vi "Eight 8-bit Ports Digital Output.vi"(2 "Packet":u64, 4 "Four 8-bit DO Ports":T1={"8-bit DO Port0"="Chassis1/Mod3/DO7:0", "8-bit DO Port1"="Chassis1/Mod3/DO7:0", "8-bit DO Port2"="Chassis1/Mod3/DO7:0", "8-bit DO Port3"="Chassis1/Mod3/DO7:0", "8-bit DO Port4"="Chassis1/Mod3/DO7:0", "8-bit DO Port5"="Chassis1/Mod3/DO7:0", "8-bit DO Port6"="Chassis1/Mod3/DO7:0", "8-bit DO Port7"="Chassis1/Mod3/DO7:0"}) -> ()   [LabVIEW 2009]
uses:
  <vilib>/eio/EIONode/EIONode.xnode
  <vilib>/rvi/eio/nirviEIOImplementation/nirviEIOImplementation.xnode
  <vilib>/rvi/eio/common/nirviEmuTemplateMethod_noerrors.vi
  <vilib>/rvi/eio/common/nirviEmuClasses.ctl
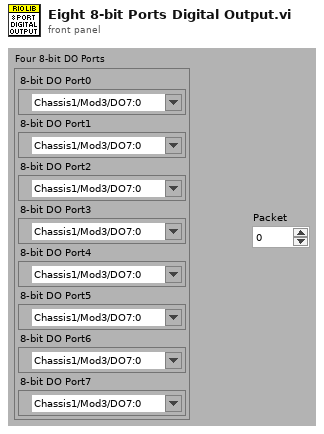
[diagram p1: front panel]
types:
  T1 = cluster{"8-bit DO Port0":refnum<k21>, "8-bit DO Port1":refnum<k21>, "8-bit DO Port2":refnum<k21>, "8-bit DO Port3":refnum<k21>, "8-bit DO Port4":refnum<k21>, "8-bit DO Port5":refnum<k21>, "8-bit DO Port6":refnum<k21>, "8-bit DO Port7":refnum<k21>}
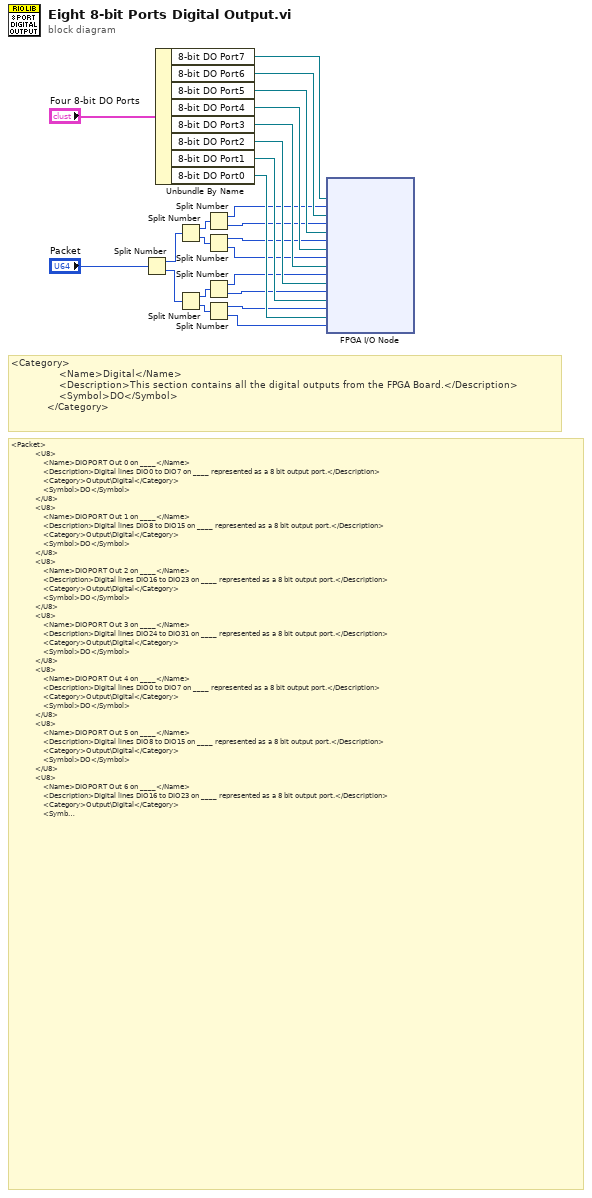
[diagram p0: block diagram]
diagram:
  # "<Packet>\n            <U8>\n                <Name>DIOPORT Out 0 on ____</Name>\n                <Description>Digital lines DIO0 to DIO7 on ____ represented as a 8 bit output port.</Description>\n                <Category>Output\\Digital</Category>\n                <Symbol>DO</Symbol>\n            </U8>\n            <U8>\n                <Name>DIOPORT Out 1 on ____</Name>\n                <Description>Digital lines DIO8 to DIO15 on ____ represented as a 8 bit output port.</Description>\n                <Category>Output\\Digital</Category>\n                <Symbol>DO</Symbol>\n            </U8>\n            <U8>\n                <Name>DIOPORT Out 2 on ____</Name>\n                <Description>Digital lines DIO16 to DIO23 on ____ represented as a 8 bit output port.</Description>\n                <Category>Output\\Digital</Category>\n                <Symbol>DO</Symbol>\n            </U8>\n            <U8>\n                <Name>DIOPORT Out 3 on ____</Name>\n                <Description>Digital lines DIO24 to DIO31 on ____ represented as a 8 bit output port.</Description>\n                <Category>Output\\Digital</Category>\n                <Symbol>DO</Symbol>\n            </U8>\n            <U8>\n                <Name>DIOPORT Out 4 on ____</Name>\n                <Description>Digital lines DIO0 to DIO7 on ____ represented as a 8 bit output port.</Description>\n                <Category>Output\\Digital</Category>\n                <Symbol>DO</Symbol>\n            </U8>\n            <U8>\n                <Name>DIOPORT Out 5 on ____</Name>\n                <Description>Digital lines DIO8 to DIO15 on ____ represented as a 8 bit output port.</Description>\n                <Category>Output\\Digital</Category>\n                <Symbol>DO</Symbol>\n            </U8>\n            <U8>\n                <Name>DIOPORT Out 6 on ____</Name>\n                <Description>Digital lines DIO16 to DIO23 on ____ represented as a 8 bit output port.</Description>\n                <Category>Output\\Digital</Category>\n                <Symbol>DO</Symbol>\n            </U8>\n            <U8>\n                <Name>DIOPORT Out 7 on ____</Name>\n                <Description>Digital lines DIO16 to DIO23 on ____ represented as a 8 bit output port.</Description>\n                <Category>Output\\Digital</Category>\n                <Symbol>DO</Symbol>\n            </U8>\n        </Packet>"
  # "<Category>\n                <Name>Digital</Name>\n                <Description>This section contains all the digital outputs from the FPGA Board.</Description>\n                <Symbol>DO</Symbol>\n            </Category>"
  n1 = Split Number(x="Packet") -> (hi(x)=w5:u32, lo(x)=w23:u32)
  n2 = Unbundle By Name("Four 8-bit DO Ports") -> ("8-bit DO Port7"=w8:refnum<k21>, "8-bit DO Port6"=w9:refnum<k21>, "8-bit DO Port5"=w10:refnum<k21>, "8-bit DO Port4"=w11:refnum<k21>, "8-bit DO Port3"=w13:refnum<k21>, "8-bit DO Port2"=w16:refnum<k21>, "8-bit DO Port1"=w19:refnum<k21>, "8-bit DO Port0"=w18:refnum<k21>)
  n3 = Split Number(x=w5) -> (hi(x)=w7:u16, lo(x)=w6:u16)
  n4 = Split Number(x=w23) -> (hi(x)=w15:u16, lo(x)=w24:u16)
  n5 = Split Number(x=w7) -> (hi(x)=w1:u8, lo(x)=w2:u8)
  n6 = Split Number(x=w6) -> (hi(x)=w3:u8, lo(x)=w4:u8)
  n7 = Split Number(x=w15) -> (hi(x)=w12:u8, lo(x)=w14:u8)
  n8 = Split Number(x=w24) -> (hi(x)=w17:u8, lo(x)=w22:u8)
  n9 = xnode "FPGA I/O Node"("I/O Item"=w1, "I/O Item"=w2, "I/O Item"=w3, "I/O Item"=w4, "I/O Item"=w12, "I/O Item"=w14, "I/O Item"=w17, "I/O Item"=w22, "FPGA I/O In"=w8, "FPGA I/O In"=w9, "FPGA I/O In"=w10, "FPGA I/O In"=w11, "FPGA I/O In"=w13, "FPGA I/O In"=w16, "FPGA I/O In"=w19, "FPGA I/O In"=w18) -> ()  [unwired: 8 out]
